vi "obtain_histogram.vi"(7 "number of bins":i32=256, 8 "error in (no error)":errorcluster, 11 "Image in":refnum<class "Image.lvclass">) -> (0 "error out":errorcluster, 2 "histogram out":cluster{i32, u32}[](graph), 3 "Image out":refnum<class "Image.lvclass">)   [LabVIEW 2010, in "Image.lvclass"]
uses:
  Image.lvclass
  ErrorController/ErrorController/class_data.vi
  <vilib>/vision/NI_Vision_Development_Module.lvlib
  ErrorController/ErrorController/ErrorController.lvclass
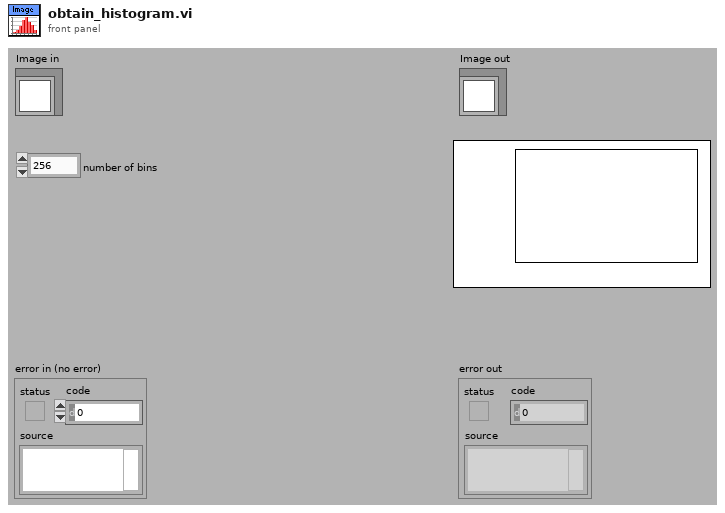
[diagram p1: front panel]
types:
  T1 = typedef "IMAQ Image.ctl" = refnum<image>
  T2 = cluster{"Starting Value":sgl, "Incremental Value":sgl, "Histogram":u32[]}
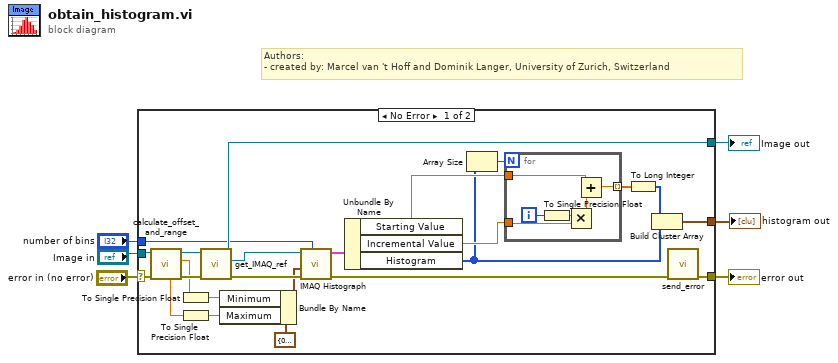
[diagram p0: block diagram]
diagram:
  # "Authors: \n- created by: Marcel van 't Hoff and Dominik Langer, University of Zurich, Switzerland"
  n1 = case shown="No Error" "error in (no error)" {
    selector: "error in (no error)" -> [w25 w38]
    tunnel: [w7 w38] -> w5
    tunnel: [w29 w37] -> w3
    tunnel: "Image in" -> [w23 w37]
    tunnel: [w26 _] -> w2
    tunnel: "number of bins" -> [w21 _]
    frame No Error {
      n2 = call-dynamic "calculate_offset_and_range.vi"("error in (no error)"=w25, "Image in"=w23) -> ("error out"=w24:errorcluster, "offset / minimum"=w17:dbl, "Image out"=w22:refnum<class "Image.lvclass">, "maximum"=w16:dbl)  [unwired: 5 in, 1 out]
      n3 = To Single Precision Float(number=w17) -> (single precision float=w10:sgl)
      n4 = To Single Precision Float(number=w16) -> (single precision float=w9:sgl)
      n5 = call-dynamic "get_IMAQ_ref.vi"("error in (no error)"=w24, "Image.lvclass in"=w22) -> ("error out"=w27:errorcluster, "Image"=w28:T1, "Image.lvclass out"=w29:refnum<class "Image.lvclass">)  [unwired: 5 in, 2 out]
      n6 = Bundle By Name(cluster=cluster{"Minimum":sgl, "Maximum":sgl} {"Minimum"=0.0, "Maximum"=0.0} ("Interval Range"), "Minimum"=w10, "Maximum"=w9) -> (w18:cluster{"Minimum":sgl, "Maximum":sgl})
      n7 = call "IMAQ Histograph"("Number of Classes"=w21, "error in (no error)"=w27, "Interval Range"=w18, "Image"=w28) -> ("error out"=w8:errorcluster, "Histogram Graph"=w30:T2)  [unwired: 4 in, 2 out]
      n8 = Unbundle By Name(w30) -> ("Starting Value"=w15:sgl, "Incremental Value"=w14:sgl, "Histogram"=w11:u32[])
      n9 = Array Size(array=w11) -> (size(s)=w12:i32)
      n10 = for {
        N: w12 -> [_]
        tunnel: [w36] -> w20 mode=indexing
        tunnel: w15 -> [w32]
        tunnel: w14 -> [w33]
        i -> [w34]
        n11 = To Single Precision Float(number=w34) -> (single precision float=w35:sgl)
        n12 = Multiply(x=w35, y=w33) -> (x*y=w31:sgl)
        n13 = Add(x=w32, y=w31) -> (x+y=w36:sgl)
      }
      n14 = To Long Integer(number=w20) -> (32bit integer=w13:i32[])
      n15 = Build Cluster Array(w13, w11) -> (w26:cluster{i32, u32}[])
      n16 = call "send_error.vi"("error in (no error)"=w8) -> ("error out"=w7:errorcluster)  [unwired: 10 in]
    }
    frame Error {
    }
  }
  "error out" <- w5
  "Image out" <- w3
  "histogram out" <- w2
